vi "Data Viewer.vi"(6 "menu options":cluster{"open":bool, "save":bool, "view":bool}={"open"=TRUE, "save"=FALSE, "view"=FALSE}, 8 "error in (no error)":errorcluster, 9 "Stop Pointer":refnum<class "Pointer.lvclass">, 10 "Framework Configuration":T1, 11 "DSF":refnum<class "Framework.lvclass">) -> (0 "error out":errorcluster)   [LabVIEW 2017, in "DSF Core.lvlib"]
uses:
  DSF Core.lvlib
  Classes/Framework/Framework.lvclass
  Typedefs/DSF Engine Framework Configuration.ctl
  Typedefs/DSF Engine Plugin Configuration.ctl
  Typedefs/DSF Timing Info.ctl
  Typedefs/DSF Engine Plugin Thread Configuration.ctl
  Typedefs/DSF Settings Info.ctl
  Typedefs/DSF Engine Transfer Group Configuration.ctl
  Typedefs/DSF Direction.ctl
  Typedefs/DSF Engine Transfer Configuration.ctl
  Typedefs/DSF Byte Order.ctl
  Typedefs/DSF Engine Channel Configuration.ctl
  Typedefs/DSF Data Type.ctl
  Typedefs/DSF Timeout Behavior.ctl
  <vilib>/NI/Memory Manager/Classes/Pointer/Pointer.lvclass
  <vilib>/NI/Memory Manager/Classes/Pointer/Pointer.lvclass/Pointer.ctl
  Classes/Framework/Framework.lvclass/Framework.ctl
  Source/Main VI/Application Data.ctl
  Source/Buffer Reader/Buffer Data.ctl
  Classes/Buffer/Buffer.lvclass
  C:/Program Files (x86)/National Instruments/LabVIEW 2017/vi.lib/NI/Memory Manager/Classes/Pointer/Pointer.lvclass
  Classes/Transfer Group Status/Status.lvclass
  Classes/Performance/Performance.lvclass/Performance.ctl
  <vilib>/NI/Memory Manager/Classes/Pointer/Read Bool.vi
  <vilib>/NI/Memory Manager/Classes/Pointer/Write Bool.vi
  <vilib>/NI/Memory Manager/Classes/Pointer/Read (No Check).vi
  <vilib>/NI/Memory Manager/Classes/Pointer/Read (No Check) Bool.vi
  <vilib>/NI/Memory Manager/Classes/Pointer/Check Move.vi
  <vilib>/NI/Memory Manager/Classes/Pointer/Write (No Check).vi
  <vilib>/NI/Memory Manager/Classes/Pointer/Write (No Check) Bool.vi
  Source/Item Tree/Get Buffer Data from Variant.vi
  <vilib>/NI/Memory Manager/Classes/Pointer/Get Size.vi
  Classes/Performance/Read Timing Status.vi
  <vilib>/NI/Memory Manager/Classes/Pointer/Check Size (0D).vi
  <vilib>/NI/Memory Manager/Classes/Pointer/Get Address.vi
  Classes/Transfer Group Status/Status Size.vi
  <vilib>/NI/Memory Manager/Classes/Pointer/Check Null Pointer.vi
  <vilib>/NI/Memory Manager/Classes/Pointer/Set Address.vi
  <vilib>/NI/Memory Manager/Classes/Pointer/Set Size.vi
  <vilib>/NI/Memory Manager/Classes/Pointer/Set Internal.vi
  <vilib>/NI/Memory Manager/Classes/Pointer/Check Count.vi
  <vilib>/NI/Memory Manager/Classes/Pointer/Check Bounds (Power of 2).vi
  Classes/Timing Status/Read Timing Status.vi
  <vilib>/NI/Memory Manager/Classes/Pointer/Errors.vi
  <vilib>/NI/Memory Manager/Classes/Pointer/Out of Bounds.vi
  <vilib>/NI/Memory Manager/Classes/Pointer/Null Pointer.vi
  <vilib>/NI/Memory Manager/Classes/Pointer/Check Bounds.vi
  Classes/Timing Status/Timing Status Size.vi
  <vilib>/NI/Memory Manager/VIs/Source.Write.String.vi
  <vilib>/NI/Memory Manager/Classes/Pointer/Write Pointer Size.vi
  <vilib>/NI/Memory Manager/Classes/Pointer/Create Error.vi
  <vilib>/NI/Memory Manager/VIs/Source.Write.Scalar.Base10.vi
  <vilib>/NI/Memory Manager/VIs/Source.Write.Scalar.Base10 (U64).vi
  <vilib>/NI/Memory Manager/Classes/Pointer/Check Pointer Bounds.vi
  <vilib>/NI/Memory Manager/Classes/Pointer/Check Buffer Bounds.vi
  <vilib>/NI/Memory Manager/VIs/New Error Cluster Constant.vi
  <vilib>/NI/Memory Manager/VIs/New Error Cluster Constant (512B).vi
  <vilib>/NI/Memory Manager/VIs/Error Cluster.Set Status.vi
  <vilib>/NI/Memory Manager/VIs/Error Cluster.Set Code.vi
  <vilib>/NI/Memory Manager/VIs/Error Cluster.Set VI Source.vi
  <vilib>/NI/Memory Manager/Constants/Constants.vi
  <vilib>/NI/Memory Manager/Constants/Library Name.vi
  <vilib>/NI/Memory Manager/Classes/Pointer/Pointer Error Info.vi
  <vilib>/NI/Memory Manager/Constants/Pointer Class Name.vi
  <vilib>/NI/Memory Manager/Classes/Pointer/Buffer Underflow.vi
  Classes/Timing Status/Timing Status.lvclass
  Classes/Configuration/Required Buffer Size (Framework).vi
  Classes/Performance/Performance.lvclass
panel:
  in  "Item Tree":string(tree)
  out "Values":string
  out "ASCII":string
  out "Late Count":u64
  out "Iteration":u64
  out "Frequency":dbl format="%.1fHz"
  out "Size":u64 format="%#_3pB"
  out "Null":bool
  out "Decimation":u64
  out "Throughput":dbl format="%_3pB/s"
  out "Hex":string
  # "Data Viewer"
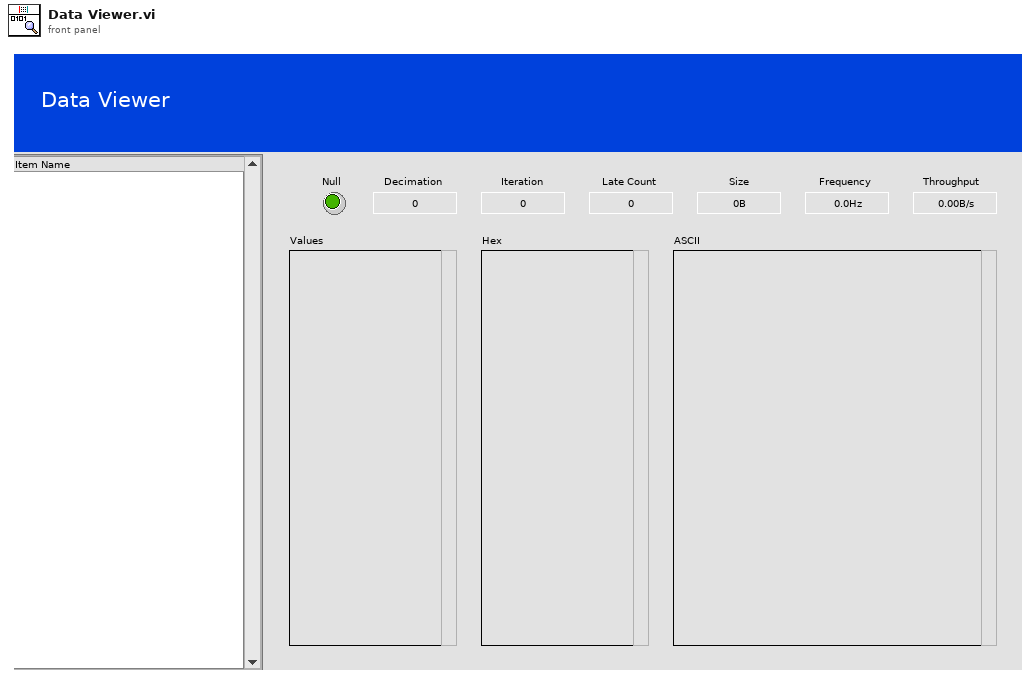
[diagram p1: front panel]
types:
  T1 = typedef "DSF Core.lvlib/DSF Engine Framework Configuration.ctl" = cluster{"Plugins":T2[]}
  T2 = typedef "DSF Core.lvlib/DSF Engine Plugin Configuration.ctl" = cluster{"name":string, "components":string[], "cycle timing":T3, "threads":T4[], "Transfer Groups":T6[], "settings":T5}
  T3 = typedef "DSF Core.lvlib/DSF Timing Info.ctl" = cluster{"priority":u64, "decimation":u64, "offset":u64}
  T4 = typedef "DSF Core.lvlib/DSF Engine Plugin Thread Configuration.ctl" = cluster{"buffer converter settings":T5, "transceiver settings":T5, "processor":i32, "priority offset":i16}
  T5 = typedef "DSF Core.lvlib/DSF Settings Info.ctl" = cluster{"key":string, "value":string}[]
  T6 = typedef "DSF Core.lvlib/DSF Engine Transfer Group Configuration.ctl" = cluster{"name":string, "direction":T7, "cycle timing":T3, "thread index":i32, "settings":T5, "Transfers":T8[], "timeout behavior":T12}
  T7 = typedef "DSF Core.lvlib/DSF Direction.ctl" = enum8{"Tx", "Rx"}
  T8 = typedef "DSF Core.lvlib/DSF Engine Transfer Configuration.ctl" = cluster{"name":string, "byte order":T9, "settings":T5, "channels":T10[]}
  T9 = typedef "DSF Core.lvlib/DSF Byte Order.ctl" = enum8{"big-endian", "little-endian"}
  T10 = typedef "DSF Core.lvlib/DSF Engine Channel Configuration.ctl" = cluster{"string offset":u64, "string data type":T11, "engine data type":T11, "name":string, "settings":T5, "units":string}
  T11 = typedef "DSF Core.lvlib/DSF Data Type.ctl" = enum8{"Bool", "SGL", "DBL", "I8", "I16", "I32", "I64", "U8", "U16", "U32", "U64"}
  T12 = typedef "DSF Core.lvlib/DSF Timeout Behavior.ctl" = enum8{"Increment Late Count", "Throw Error"}
  T13 = typedef "DSF Core.lvlib/Buffer Data.ctl" = cluster{"Buffer":refnum<class "Buffer.lvclass">, "Status":refnum<class "Status.lvclass">, "decimation":u64, "avg bandwidth":dbl, "data type":T11, "units":string, "channels":T10[], "channel":bool, "engine (T) / string (F)":bool}
  T14 = typedef "DSF Core.lvlib/Application Data.ctl" = cluster{"Item Tree Control":refnum<vi>, "Top-Level VI":refnum<vi>, "menu reference":refnum<k9>, "Framework":refnum<class "Framework.lvclass">, "buffer queue":refnum<queue>, "Stop Pointer":refnum<class "Pointer.lvclass">, "Buffer Variant":variant, "Framework Configuration":T1}
  T15 = typedef "DSF Core.lvlib/Status.lvclass/Status Data.ctl" = cluster{"late count":u64, "iteration":u64, "duration":u32}
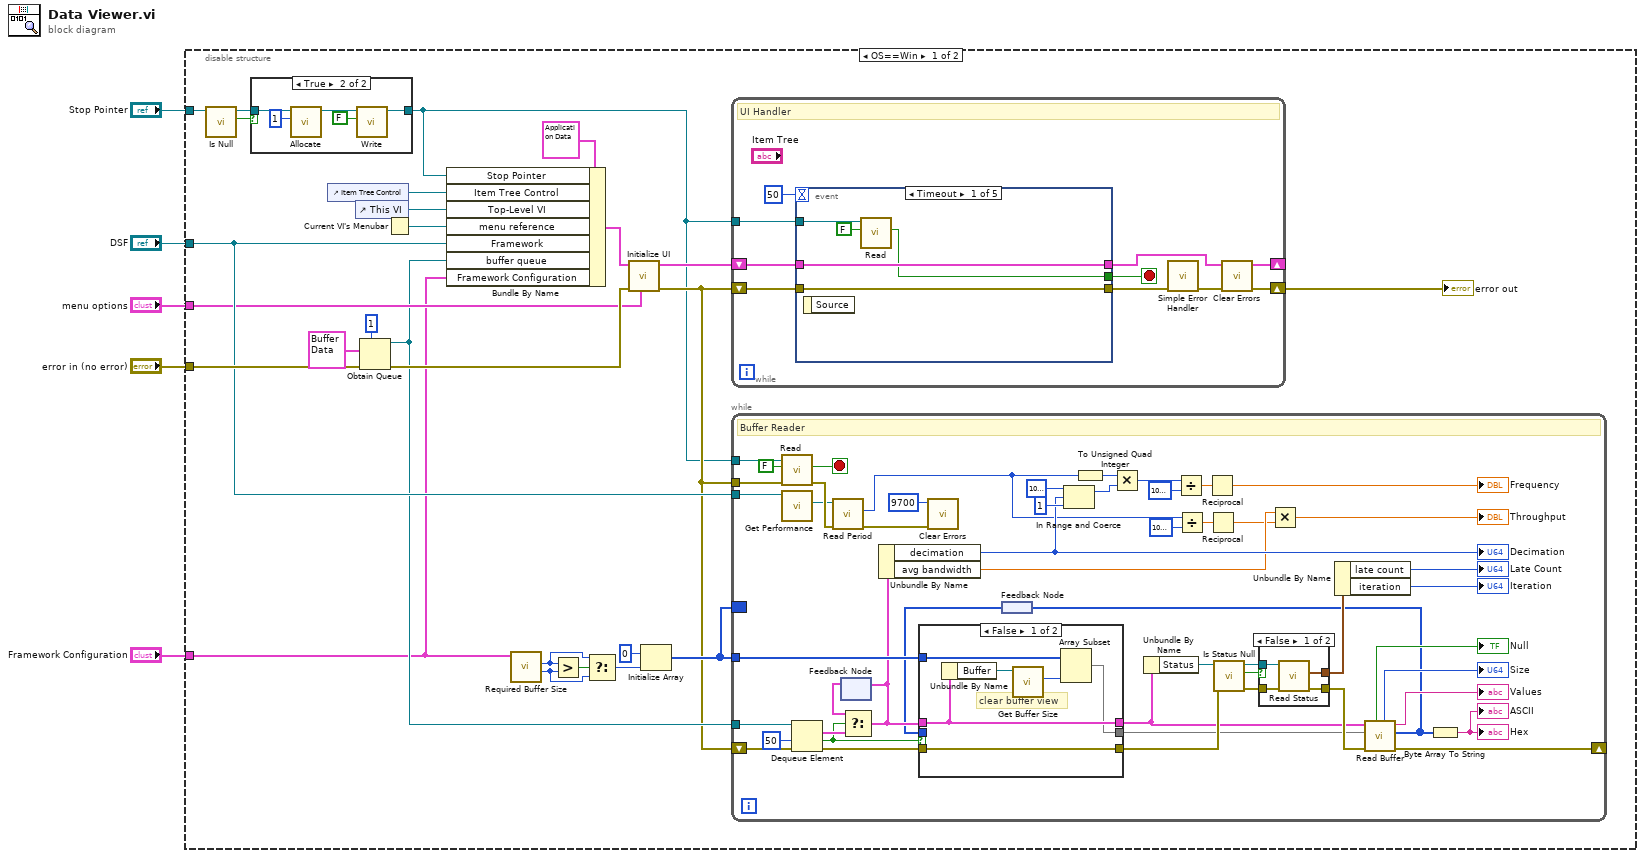
[diagram p0: block diagram]
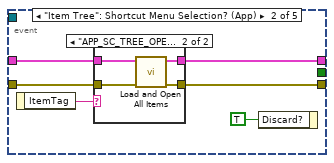
[diagram p5: hidden frame]
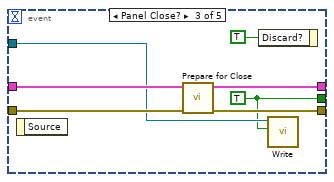
[diagram p7: hidden frame]
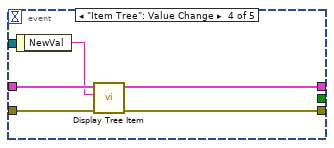
[diagram p8: hidden frame]
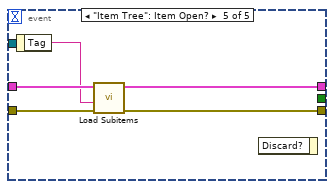
[diagram p9: hidden frame]
diagram:
  n1 = disable-structure shown="OS==Win" {
    disable-tunnel: "error in (no error)" -> [w24 _]
    disable-tunnel: "Stop Pointer" -> [w17 _]
    disable-tunnel: "DSF" -> [w15 _]
    disable-tunnel: "menu options" -> [w11 _]
    disable-tunnel: "Framework Configuration" -> [w8 _]
    frame condition #0 (active) {
      n2 = call <vilib>:"Is Null.vi"("Pointer in"=w17) -> ("null?"=w16:bool)  [unwired: 8 in, 2 out]
      n3 = case shown="True" w16 {
        tunnel: [w31 w33] -> w6
        tunnel: w17 -> [w31 w35]
        frame False {
        }
        frame True {
          n4 = call <vilib>:"Allocate.vi"("size"=u64 1, "Pointer in"=w35) -> ("Pointer out"=w34:refnum<class "Pointer.lvclass">)  [unwired: 8 in, 1 out]
          n5 = call-poly <vilib>:"Write.vi"("value"=FALSE ("buffer in"), "Pointer in"=w34) -> ("Pointer out"=w33:refnum<class "Pointer.lvclass">)  [unwired: 6 in, 3 out]
        }
      }
      n6 = control-ref of="Item Tree Control"() -> (w26:refnum<vi>)
      n7 = control-ref of="This VI"() -> (w29:refnum<vi>)
      n8 = Obtain Queue(max queue size (-1, unlimited)=1, element data type=T13 {"Buffer"=refnum, "Status"=refnum, "decimation"=0, "avg bandwidth"=0.0, "data type"=enum."Bool", "units"="", "channels"=[], "channel"=FALSE, "engine (T) / string (F)"=FALSE} ("Buffer data"), error in (no error)=w24) -> (queue out=w10:refnum<queue>, error out=w23:errorcluster)  [unwired: 2 in, 1 out]
      n9 = Current VI's Menubar() -> (w27:refnum<k9>)
      n10 = Bundle By Name(cluster=T14 {"Item Tree Control"=refnum, "Top-Level VI"=refnum, "menu reference"=refnum, "Framework"=refnum, "buffer queue"=refnum, "Stop Pointer"=refnum, "Buffer Variant"=variant, "Framework Configuration"={"Plugins"=[]}}, "Stop Pointer"=w6, "Item Tree Control"=w26, "Top-Level VI"=w29, "menu reference"=w27, "Framework"=w15, "buffer queue"=w10, "Framework Configuration"=w8) -> (w9:T14)
      n11 = call-poly "Required Buffer Size.vi"("Framework Configuration in"=w8) -> ("total engine buffer size"=w12:u64, "total string buffer size"=w13:u64)  [unwired: 7 in, 2 out]
      n12 = Greater?(x=w13, y=w12) -> (0:w22:bool)
      n13 = Select(t=w13, s=w22, f=w12) -> (s? t:f=w20:u64)
      n14 = call "Initialize UI.vi"("menu options"=w11, "error in (no error)"=w23, "Application Data in"=w9) -> ("error out"=w7:errorcluster, "Application Data out"=w19:T14)  [unwired: 7 in]
      n15 = Initialize Array(u8 0 ("element"), w20) -> (w14:u8[])
      n16 = while {
        shift-right: [w106] -> w28
        shift-left: w7 -> [w110]
        shift-right: [w107] -> _
        shift-left: w19 -> [w105]
        tunnel: w6 -> [w103]
        stop <- w104 stop-if-true
        # "UI Handler"
        n17 = event shown="[0] Timeout" {
          selector: _ -> [_ _ _ _ _]
          dyn-events: _ -> [_ _ _ _ _]
          timeout: 50 -> [_ _ _ _ _]
          tunnel: [w111 _ w128 _ _] -> w104
          tunnel: w110 -> [w115 w118 w134 w139 w144]
          tunnel: [w115 w119 w132 w138 w143] -> w108
          tunnel: w105 -> [w114 w120 w130 w136 w142]
          tunnel: [w114 w116 w131 w137 w141] -> w107
          tunnel: w103 -> [w113 _ w129 _ _]
          event Timeout {
            n18 = event-data() -> ()  [unwired: 1 in, 1 out]
            n19 = call-poly <vilib>:"Read.vi"("value in"=FALSE ("buffer in"), "Pointer in"=w113) -> ("value out"=w111:bool)  [unwired: 6 in, 3 out]
          }
          event "Item Tree": Shortcut Menu Selection? (App) {
            n20 = event-data() -> ("ItemTag"=w121:string)  [unwired: 1 in]
            n21 = case shown="\"APP_SC_TREE_OPEN_ALL_ITEMS\"" w121 {
              tunnel: w120 -> [w122 w127]
              tunnel: [w123 w125] -> w119
              tunnel: w118 -> [w123 w126]
              tunnel: [w122 w124] -> w116
              frame Default {
              }
              frame "APP_SC_TREE_OPEN_ALL_ITEMS" {
                n22 = call "Load and Open All Items.vi"("error in (no error)"=w126, "Application Data in"=w127) -> ("error out"=w125:errorcluster, "Application Data out"=w124:T14)  [unwired: 8 in]
              }
            }
            n23 = event-data("Discard?"=TRUE) -> ()  [unwired: 1 in, 1 out]
          }
          event Panel Close? {
            w128 = TRUE
            n24 = event-data() -> ()  [unwired: 1 in, 1 out]
            n25 = call "Prepare for Close.vi"("error in (no error)"=w134, "Application Data in"=w130) -> ("error out"=w132:errorcluster, "Application Data out"=w131:T14)  [unwired: 8 in]
            n26 = event-data("Discard?"=TRUE) -> ()  [unwired: 1 in, 1 out]
            n27 = call-poly <vilib>:"Write.vi"("value"=w128, "Pointer in"=w129) -> ()  [unwired: 6 in, 4 out]
          }
          event "Item Tree": Value Change {
            n28 = event-data() -> ("NewVal"=w135:string)  [unwired: 1 in]
            n29 = call "Display Tree Item.vi"("error in (no error)"=w139, "Tag"=w135, "Application Data in"=w136) -> ("error out"=w138:errorcluster, "Application Data out"=w137:T14)  [unwired: 7 in]
          }
          event "Item Tree": Item Open? {
            n30 = event-data() -> ("Tag"=w140:string)  [unwired: 1 in]
            n31 = call "Load Subitems.vi"("error in (no error)"=w144, "Tag"=w140, "Application Data in"=w142) -> ("error out"=w143:errorcluster, "Application Data out"=w141:T14)  [unwired: 6 in, 1 out]
            n32 = event-data() -> ()  [unwired: 2 in, 1 out]
          }
        }
        n33 = call <vilib>:"Simple Error Handler.vi"("error in (no error)"=w108) -> ("error out"=w109:errorcluster)  [unwired: 4 in, 4 out]
        n34 = call <vilib>:"Clear Errors.vi"("error in (no error)"=w109) -> ("error out"=w106:errorcluster)  [unwired: 5 in, 1 out]
      }
      "error out" <- w28
      n35 = while {
        tunnel: w10 -> [w86]
        shift-right: [w43] -> _
        shift-left: w7 -> [w83]
        tunnel: w14 -> [w74]
        tunnel: w6 -> [w78]
        tunnel: w15 -> [w57]
        border: w14 -> [_]
        tunnel: w7 -> [w48]
        stop <- w79 stop-if-true
        # "Buffer Reader"
        n36 = call-poly <vilib>:"Read.vi"("error in (no error)"=w48, "value in"=FALSE ("buffer in"), "Pointer in"=w78) -> ("error out"=w47:errorcluster, "value out"=w79:bool)  [unwired: 5 in, 2 out]
        n37 = call "Get Performance.vi"("Framework in"=w57) -> ("Performance"=w46:refnum<class "Performance.lvclass">)  [unwired: 9 in, 1 out]
        n38 = Dequeue Element(queue=w86, timeout in ms (-1)=50, error in (no error)=w83) -> (element=w84:T13, timed out?=w75:bool, error out=w87:errorcluster)  [unwired: 1 out]
        n39 = call "Read Period.vi"("error in (no error)"=w47, "Framework Performance in"=w46) -> ("error out"=w68:errorcluster, "period"=w51:u32)  [unwired: 7 in, 1 out]
        n40 = feedback #1() -> (w73:T13)  [unwired: 1 in]
        n41 = Select(t=w73, s=w75, f=w84) -> (s? t:f=w70:T13)
        n42 = feedback-in #1(w70) -> ()
        n43 = Unbundle By Name(w70) -> ("decimation"=w55:u64, "avg bandwidth"=w50:dbl)
        "Decimation" <- w55
        n44 = call <vilib>:"Clear Errors.vi"("error in (no error)"=w68, "specific error code to clear (0: all)"=9700) -> ()  [unwired: 4 in, 2 out]
        n45 = feedback #2() -> (w59:u8[])
        n46 = case shown="False" w75 {
          tunnel: w59 -> [_ w101]
          tunnel: w70 -> [w94 w100]
          tunnel: w74 -> [w98 _]
          tunnel: [w93 w101] -> w39
          tunnel: w87 -> [w95 w99]
          tunnel: [w94 w100] -> w38
          tunnel: [w95 w99] -> w64
          frame False {
            # "clear buffer view"
            n47 = Unbundle By Name(w94) -> ("Buffer"=w96:refnum<class "Buffer.lvclass">)
            n48 = call "Get Buffer Size.vi"("Buffer in"=w96) -> ("buffer size"=w97:u64)  [unwired: 9 in, 1 out]
            n49 = Array Subset(array=w98, length=w97) -> (w93:u8[])  [unwired: 1 in]
          }
          frame True {
          }
        }
        n50 = In Range and Coerce(upper limit=u64 1000000000, x=w55, lower limit=u64 1) -> (coerced(x)=w54:u64)  [unwired: 1 out]
        n51 = To Unsigned Quad Integer(1:w51) -> (0:w72:u64)
        n52 = Multiply(x=w72, y=w54) -> (x*y=w82:u64)
        n53 = Unbundle By Name(w38) -> ("Status"=w67:refnum<class "Status.lvclass">)
        n54 = Divide(x=w82, y=u64 1000000) -> (x/y=w71:dbl)
        n55 = Divide(x=w51, y=u64 1000000) -> (x/y=w52:dbl)
        n56 = Reciprocal(x=w71) -> (1/x=→"Frequency":dbl)
        n57 = Reciprocal(x=w52) -> (1/x=w49:dbl)
        n58 = call "Is Status Null.vi"("error in (no error)"=w64, "status pointer in"=w67) -> ("error out"=w65:errorcluster, "null?"=w63:bool, "status pointer out"=w66:refnum<class "Status.lvclass">)  [unwired: 7 in]
        n59 = case shown="False" w63 {
          tunnel: [w91 w92] -> w44
          tunnel: w66 -> [w90 _]
          tunnel: w65 -> [w89 w92]
          tunnel: [w88 _] -> w62
          frame False {
            n60 = call "Read Status.vi"("error in (no error)"=w89, "status pointer in"=w90) -> ("error out"=w91:errorcluster, "status"=w88:T15)  [unwired: 7 in, 1 out]
          }
          frame True {
          }
        }
        n61 = Multiply(x=w50, y=w49) -> (x*y=→"Throughput":dbl)
        n62 = Unbundle By Name(w62) -> ("late count"=→"Late Count":u64, "iteration"=→"Iteration":u64)
        n63 = call "Read Buffer.vi"("error in (no error)"=w44, "buffer in"=w39, "Buffer data"=w38) -> ("error out"=w43:errorcluster, "buffer out"=w37:u8[], "buffer string"=→"Values":string, "buffer size"=→"Size":u64, "null?"=→"Null":bool)  [unwired: 4 in]
        n64 = feedback-in #2(w37) -> ()
        n65 = Byte Array To String(unsigned byte array=w37) -> (string=→"Hex" →"ASCII":string)
      }
    }
    frame condition #1 {
    }
  }
